vi "Write User system setting file.vi"(10 "User system setting file":T1, 11 "Test Framework in":refnum<class "Test Framework.lvclass">) -> (3 "Test Framework out":refnum<class "Test Framework.lvclass">)   [LabVIEW 2020, in "Test Framework.lvclass"]
uses:
  Test Framework.lvclass
  Test Framework.lvclass/Test Framework.ctl
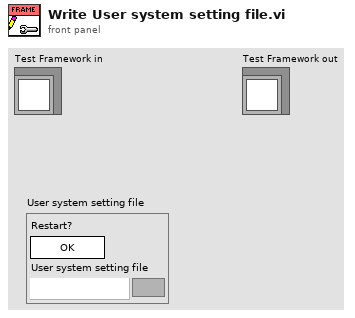
[diagram p1: front panel]
types:
  T1 = cluster{"Restart?":bool, "User system setting file":path}
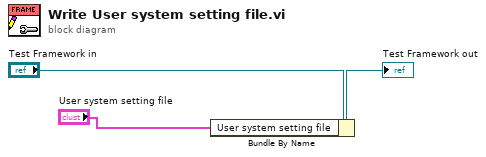
[diagram p0: block diagram]
diagram:
  n1 = Bundle By Name(cluster="Test Framework in", "User system setting file"="User system setting file") -> (→"Test Framework out":refnum<class "Test Framework.lvclass">)
